vi "CalDiaVelAll.vi"() -> ()   [LabVIEW 2017]
uses:
  <vilib>/Utility/file.llb/Write To Spreadsheet File (string).vi
  <vilib>/Utility/file.llb/Write To Spreadsheet File (DBL).vi
panel:
  in  "Calibration (1 pixel = ?um)":dbl=1.45
  out "Measurment Progress":u8(slide) scale=0.0..36.0
  out "Quantifying":dbl
  out "Total Video Segments to Quantify":dbl
  # "This VI performs diameter and velocity measurements of all videos in the selected folder. The user is prompted to select the folder after which they choose a point on the top vessel wall for all the segments then a point on the bottom vessel wall. The VI then runs through all the segments and outputs the values into two text files 'Diameter' and 'Velocity'. Due to dependencies this VI is currently set to use frame 5000 as a template"
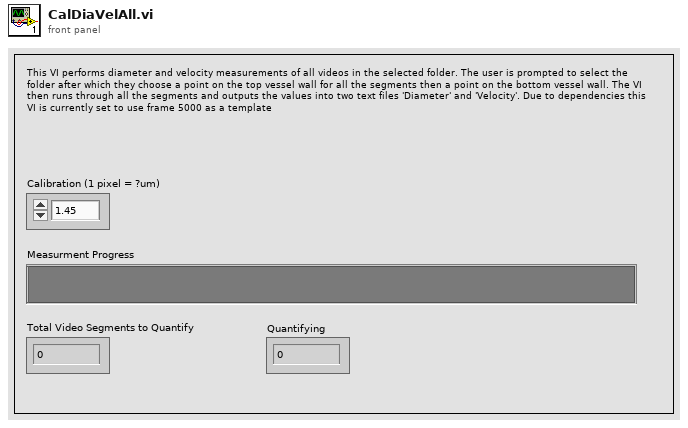
[diagram p1: front panel]
types:
  T1 = typedef "IMAQ AVI2 Refnum.ctl" = refnum<k20>
  T2 = typedef "IMAQ Image.ctl" = refnum<image>
  T3 = typedef "IMAQ Point" = cluster{"X":sgl, "Y":sgl}
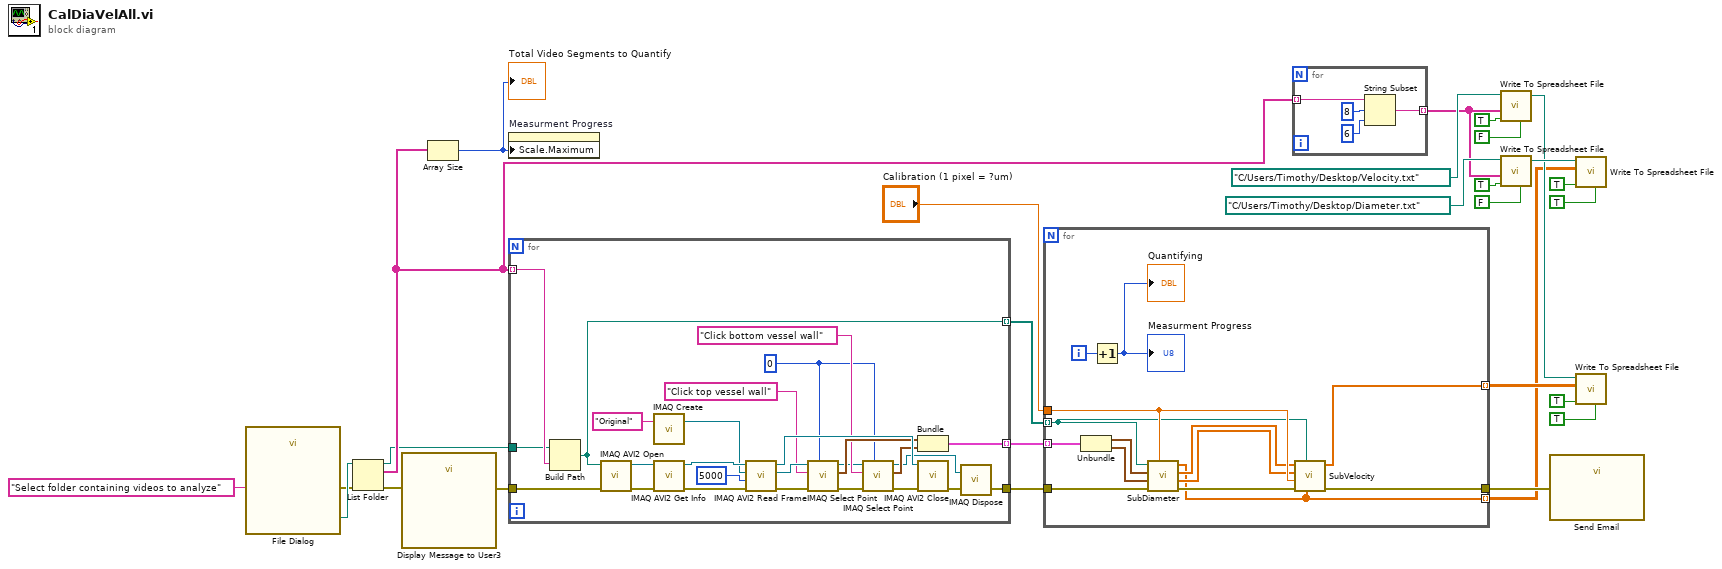
[diagram p0: block diagram]
diagram:
  n1 = call "File Dialog"("prompt"="Select folder containing videos to analyze") -> ("selected path"=w27:path, "error out"=w26:errorcluster)  [unwired: 11 in, 2 out]
  n2 = List Folder(path=w27, error in=w26) -> (path out=w4:path, filenames=w5:string[], error out=w7:errorcluster)  [unwired: 2 in, 1 out]
  n3 = call "Display Message to User3"("error in (no error)"=w7) -> ("error out"=w6:errorcluster)  [unwired: 9 in, 1 out]
  n4 = Array Size(array=w5) -> (size(s)=w25:i32)
  "Total Video Segments to Quantify" <- w25
  n5 = property on="Measurment Progress" class="Slide (strict)"("Scale.Maximum"=w25) -> ()  [unwired: 2 in, 2 out]
  n6 = for {
    tunnel: [w44] -> w9
    tunnel: [w46] -> w8 mode=indexing
    tunnel: [w36] -> w10 mode=indexing
    tunnel: w6 -> [w31]
    tunnel: w5 -> [w30] mode=indexing
    tunnel: w4 -> [w29]
    w32 = 0 ("Window Number (0...15)")
    n7 = Build Path(base path=w29, name or relative path=w30) -> (appended path=w46:path)
    n8 = call "IMAQ AVI2 Open"("error in (no error)"=w31, "AVI File Path"=w46) -> ("error out"=w53:errorcluster, "AVI Refnum"=w54:T1)  [unwired: 8 in]
    n9 = call "IMAQ Create"("Image Name"="Original") -> ("New Image"=w50:T2)  [unwired: 4 in, 1 out]
    n10 = call "IMAQ AVI2 Get Info"("error in (no error)"=w53, "AVI Refnum"=w54) -> ("error out"=w49:errorcluster, "AVI Refnum (duplicate)"=w52:T1)  [unwired: 5 in, 3 out]
    n11 = call "IMAQ AVI2 Read Frame"("error in (no error)"=w49, "Frame Number"=u32 5000, "Image"=w50, "AVI Refnum"=w52) -> ("error out"=w43:errorcluster, "Image Out"=w42:T2, "AVI Refnum (duplicate)"=w47:T1)  [unwired: 5 in]
    n12 = call "IMAQ Select Point"("Window Number (0...15)"=w32, "error in (no error)"=w43, "Prompt"="Click top vessel wall", "Image In"=w42) -> ("error out"=w40:errorcluster, "Point"=w37:T3, "Image Out (duplicate)"=w33:T2)  [unwired: 4 in, 1 out]
    n13 = call "IMAQ Select Point"("Window Number (0...15)"=w32, "error in (no error)"=w40, "Prompt"="Click bottom vessel wall", "Image In"=w33) -> ("error out"=w39:errorcluster, "Point"=w38:T3, "Image Out (duplicate)"=w34:T2)  [unwired: 4 in, 1 out]
    n14 = Bundle("Point"=w37, "Point"=w38) -> (w36:cluster{"Point":T3, "Point":T3})  [unwired: 1 in]
    n15 = call "IMAQ AVI2 Close"("error in (no error)"=w39, "AVI Refnum"=w47) -> ("error out"=w45:errorcluster)  [unwired: 9 in]
    n16 = call "IMAQ Dispose"("Image"=w34, "error in (no error)"=w45) -> ("error out"=w44:errorcluster)  [unwired: 4 in]
  }
  n17 = for {
    tunnel: w9 -> [w68]
    tunnel: "Calibration (1 pixel = ?um)" -> [w65]
    tunnel: w10 -> [w61] mode=indexing
    tunnel: w8 -> [w58] mode=indexing
    tunnel: [w57] -> w3
    tunnel: [w56] -> w2 mode=indexing
    tunnel: [w55] -> w1 mode=indexing
    i -> [w67]
    n18 = Unbundle(w61) -> ("Point"=w60:T3, "Point"=w59:T3)
    n19 = Increment(x=w67) -> (x+1=→"Quantifying" →"Measurment Progress":i32)
    n20 = call "SubDiameter.vi"("Calibration (1 pixel = ?um)"=w65, "error in (no error)"=w68, "Bot Wall"=w59, "Top wall"=w60, "AVI Path"=w58) -> ("error out"=w62:errorcluster, "Y Mid"=w63:sgl[], "X Mid"=w64:sgl[], "Diameter"=w55:dbl[])  [unwired: 3 in]
    n21 = call "SubVelocity.vi"("Vessel Diameter"=w55, "AVI Path"=w58, "error in (no error)"=w62, "Calibration factor (1 pix = ? um)"=w65, "Y"=w63, "X"=w64) -> ("error out"=w57:errorcluster, "Velocity"=w56:dbl[])  [unwired: 2 in]
  }
  n22 = for {
    tunnel: w5 -> [w72] mode=indexing
    tunnel: [w69] -> w11 mode=indexing
    n23 = String Subset(string=w72, offset (0)=8, length (rest)=6 ("length (rest)")) -> (substring=w69:string)
  }
  n24 = call-poly <vilib>:"Write To Spreadsheet File.vi"("transpose? (no:F)"=FALSE, "append to file? (new file:F)"=TRUE, "1D data"=w11, "file path (dialog if empty)"=path "C:/Users/Timothy/Desktop/Velocity.txt") -> ("new file path (Not A Path if cancelled)"=w12:path)  [unwired: 4 in]
  n25 = call-poly <vilib>:"Write To Spreadsheet File.vi"("transpose? (no:F)"=FALSE, "append to file? (new file:F)"=TRUE, "1D data"=w11, "file path (dialog if empty)"=path "C:/Users/Timothy/Desktop/Diameter.txt") -> ("new file path (Not A Path if cancelled)"=w16:path)  [unwired: 4 in]
  n26 = call "Send Email"("error in"=w3) -> ()  [unwired: 10 in, 1 out]
  n27 = call-poly <vilib>:"Write To Spreadsheet File.vi"("transpose? (no:F)"=TRUE, "append to file? (new file:F)"=TRUE, "2D data"=w1, "file path (dialog if empty)"=w16) -> ()  [unwired: 4 in, 1 out]
  n28 = call-poly <vilib>:"Write To Spreadsheet File.vi"("transpose? (no:F)"=TRUE, "append to file? (new file:F)"=TRUE, "2D data"=w2, "file path (dialog if empty)"=w12) -> ()  [unwired: 4 in, 1 out]
